vi "Analog Trigger.vi"() -> ()   [LabVIEW 2025]
doc: "Analog Trigger Example\n\nThis example opens a trigger on an analog channel with the upper and lower bound supplied by the user on the front panel. It will display the most recent bounds violation as well as whether the analog channel is currently in bounds. \n\nThis example expects a USB cable connected from your development PC to the Type B USB Jack (next to the power input) on the roboRIO."
uses:
  <vilib>/Rock Robotics/SystemInterfaces/AI/FPGA_AIChannel.ctl
  <vilib>/Rock Robotics/WPI/AnalogTrigger/WPI_AnalogTriggerOpen_Analog.vi
panel:
  out "In Bounds":bool
  out "Upper Trigger":bool
  in  "Channel":T1=enum."AI 1"
  out "Lower Trigger":bool
  in  "Lower Trigger Limit":dbl=2.0
  in  "Upper Trigger Limit":dbl=4.0
  in  "stop":bool
  # "Set these inputs before running."
  # "Output information."
  # "Boolean LEDS will display the most recent trigger and whether the analog value is currently in bounds."
  # "This shows wiring for a typical analog input using a potentiometer.  In this case the potentiometer is being powered with 5 volts, and the Signal returned will vary from 0 to 5 volts"
  # "potentiometer"
  # "Gnd"
  # "S"
  # "V"
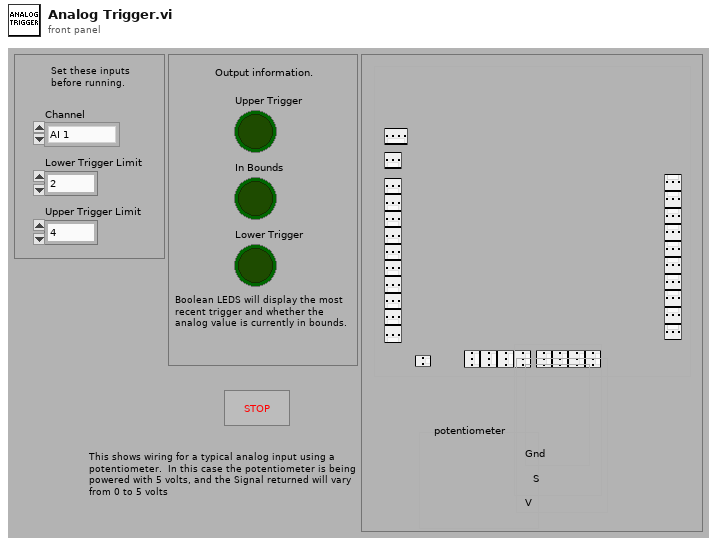
[diagram p1: front panel]
types:
  T1 = typedef "FPGA_AIChannel.ctl" = enum8{"AI 0", "AI 1", "AI 2", "AI 3", "AI MXP 0", "AI MXP 1", "AI MXP 2", "AI MXP 3", "Invalid"}
  T2 = typedef "WPI_AnalogChannelDevRef.ctl" = cluster{"DevStatus":errorcluster, "Analog Channel":T1}
  T3 = typedef "FPGA_AnalogTriggerDevRef.ctl" = cluster{"DevStatus":errorcluster, "AnalogTriggerIndex":T4}
  T4 = typedef "FPGA_AnalogTriggerIndex.ctl" = enum8{"Trig 0", "Trig 1", "Trig 2", "Trig 3", "Trig 4", "Trig 5", "Trig 6", "Trig 7", "Invalid"}
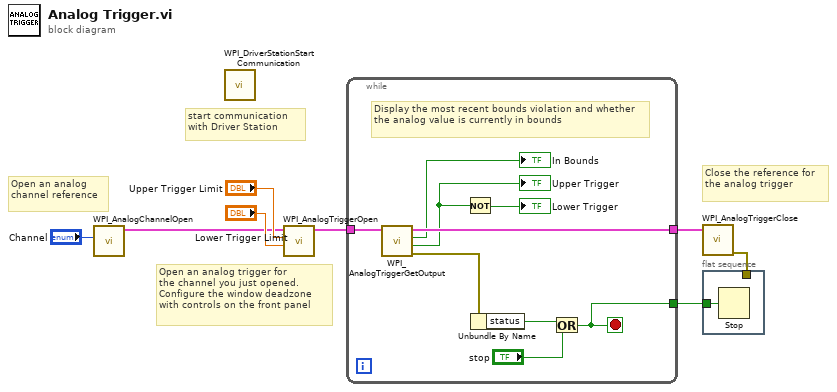
[diagram p0: block diagram]
diagram:
  # "start communication with Driver Station"
  # "Open an analog channel reference"
  # "Close the reference for \nthe analog trigger"
  # "Open an analog trigger for\nthe channel you just opened.\nConfigure the window deadzone\nwith controls on the front panel"
  n1 = call <vilib>:"WPI_AnalogChannelOpen.vi"("Analog Channel"="Channel") -> ("AIDeviceRef"=w3:T2)  [unwired: 2 in, 8 out]
  n2 = call <vilib>:"WPI_DriverStationStart Communication.vi"() -> ()  [unwired: 3 in, 9 out]
  n3 = call-poly <vilib>:"WPI_AnalogTriggerOpen.vi"("LowerLimit (v)"="Lower Trigger Limit", "UpperLimit (v)"="Upper Trigger Limit", "AnalogTriggerSource"=w3) -> ("AnalogTriggerDevRef"=w8:T3)  [unwired: 7 in, 1 out]
  n4 = while {
    tunnel: w8 -> [w17]
    tunnel: [w16] -> w5
    tunnel: [w9] -> w2
    stop <- w9 stop-if-true
    # "Display the most recent bounds violation and whether the analog value is currently in bounds"
    n5 = call <vilib>:"WPI_AnalogTriggerGetOutput.vi"("AnalogTriggerDevRef"=w17) -> ("error out"=w11:errorcluster, "Trigger State"=w13:bool, "In Window"=→"In Bounds":bool, "AnalogTriggerDevRef"=w16:T3)  [unwired: 1 in, 6 out]
    "Upper Trigger" <- w13
    n6 = Not(x=w13) -> (.not. x?=→"Lower Trigger":bool)
    n7 = Unbundle By Name(w11) -> ("status"=w12:bool)
    n8 = Or(x=w12, y="stop") -> (x .or. y?=w9:bool)
  }
  n9 = call <vilib>:"WPI_AnalogTriggerClose.vi"("AnalogTriggerDevRef"=w5) -> ("error out"=w1:errorcluster)  [unwired: 2 in, 8 out]
  n10 = flat-sequence {
    tunnel: w2 -> [w18]
    tunnel: w1 -> [_]
    frame #0 {
      n11 = Stop(stop? (T)=w18) -> ()
    }
  }
